vi "Accept.vi"(8 "error in (no error)":errorcluster, 10 "EquipmentVisitor":refnum<class "EquipmentVisitor.lvclass">, 11 "reference in":refnum<class "Laser.lvclass">) -> (0 "error out":errorcluster, 3 "reference in":refnum<class "Laser.lvclass">)   [LabVIEW 2012]
uses:
  EquipmentVisitor_class/EquipmentVisitor.lvclass
  Laser.lvclass
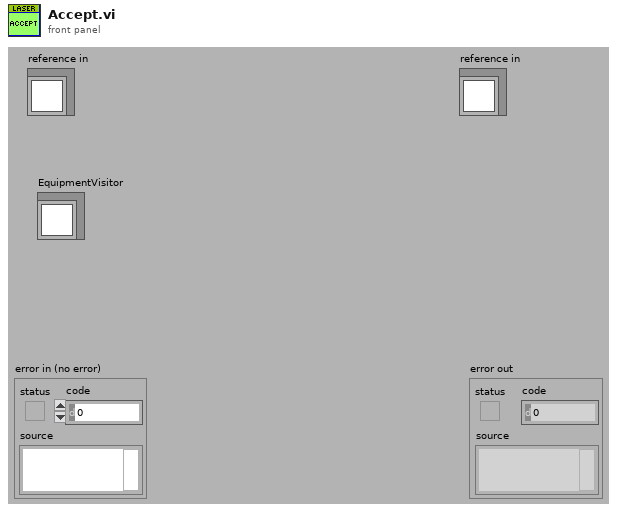
[diagram p1: front panel]
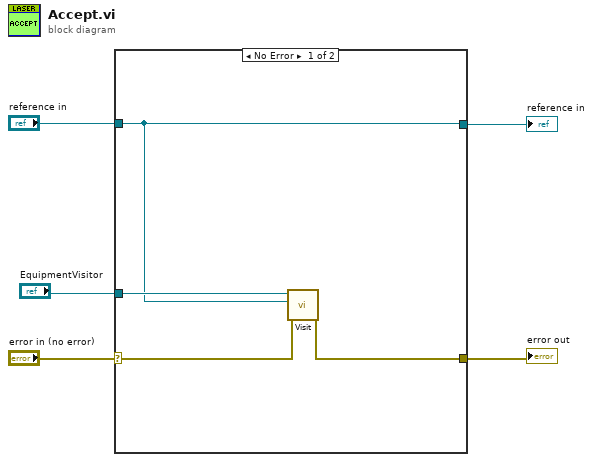
[diagram p0: block diagram]
diagram:
  n1 = case shown="No Error" "error in (no error)" {
    selector: "error in (no error)" -> [w7 w11]
    tunnel: [w6 w11] -> w4
    tunnel: [w8 w10] -> w2
    tunnel: "reference in" -> [w8 w10]
    tunnel: "EquipmentVisitor" -> [w9 _]
    frame No Error {
      n2 = call-dynamic "Visit.vi"("error in (no error)"=w7, "Equipment"=w8, "reference in"=w9) -> ("error out"=w6:errorcluster)  [unwired: 7 in, 1 out]
    }
    frame Error {
    }
  }
  "error out" <- w4
  "reference in" <- w2
